vi "FPGA VI_Simulated.vi"() -> ()   [LabVIEW 2015]
uses:
  Types/Injector.Timing.ctl
  Types/Injection.Core.Settings.ctl
  Types/Injection.Global.Settings.ctl
  <vilib>/Platform/TimedLoop/XDataNode/timing_clust.ctl
  <vilib>/Platform/TimedLoop/XDataNode/nitl_modes.ctl
  <vilib>/Platform/TimedLoop/XDataNode/wakeup.ctl
  Types/Injection.Core.Internal.Settings.ctl
  <vilib>/rvi/DataTransferAndStorage/Container/Common/niFpgaContainerGetUniqueNameForEmu.vi
  <vilib>/rvi/DataTransferAndStorage/Container/Common/niFpgaContainerSetEmuInfo.vi
  <vilib>/rvi/eio/common/nirviEmuReportErrorAndStop.vi
  <vilib>/rvi/Emulation/niFpgaGetClockAttributes.vi
  <vilib>/rvi/Emulation/niFpgaSctlEmulationGetInTimedLoop.vi
  <vilib>/rvi/Emulation/niFpgaEmulationReportErrorSimple.vi
  <vilib>/rvi/Memory/Memory_Emulation/nirvimemoryFastEmulation.vi
  <vilib>/rvi/Memory/Memory_Emulation/nirvimemoryEmulation.vi
  <vilib>/rvi/Emulation/niFpgaEmulationIsFPGAContextNoSignature.vi
  <vilib>/rvi/Emulation/niFpgaProcessEmulError.vi
  <vilib>/rvi/errors/nirviReportUnexpectedCaseInternalError (U32).vi
  <vilib>/rvi/Emulation/niFpgaCriticalErrorInLSC.vi
  <vilib>/rvi/DataTransferAndStorage/Container/Common/niFpgaContainerExecOnDevCompGetState.vi
  <vilib>/rvi/errors/niFpgaSetErrorForExecOnDevCompSimple.vi
  <vilib>/rvi/FIFO/Fifo_Resource/nirvififoEmulationSetSize.vi
  <vilib>/rvi/FIFO/Fifo_Resource/nirviFifoEmulationQueueMgr.vi
  <instcachedir>/0/nirviFifoEmulationQueueMgr_E5CAEC123FF24DC58D834DCA3CDAA9B5.lvgen/nirviFifoEmulationQueueMgr_E5CAEC123FF24DC58D834DCA3CDAA9B5_010.vi
  <vilib>/rvi/FIFO/Fifo_Resource/nirvififoEmulationDetermineInputValidOut.vi
  <vilib>/rvi/FIFO/Fifo_Resource/nirvififoEmulationCreateLock.vi
  <vilib>/rvi/FIFO/Fifo_Resource/nirvififoEmulationObtainLock.vi
  <vilib>/rvi/FIFO/Fifo_Resource/nirvififoEmulationReleaseLock.vi
  <vilib>/rvi/occurrence/nirviWaitOnOccurrenceBase.vi
  <vilib>/rvi/errors/nirviReportUnexpectedCaseInternalError.vi
  <vilib>/Utility/error.llb/Clear Errors.vi
  <vilib>/rvi/interface/RandomDataEmulation/niFpgaRandomDataHandleErrors.vi
  <instcachedir>/0/nirviFifoEmulationQueueMgr_E5CAEC123FF24DC58D834DCA3CDAA9B5.lvgen/nirviFifoEmulationQueueMgr_E5CAEC123FF24DC58D834DCA3CDAA9B5_008.vi
  <vilib>/rvi/LocalResourceManager/LocalResourceManager.xnode
  <vilib>/rvi/DataTransferAndStorage/Container/XNode/niFpgaContainer.xnode
  <vilib>/Platform/TimedLoop/XDataNode/XDataNode.xnode
  <vilib>/rvi/FIFO/Fifo_Resource/niFpgaFifoEmulationRefIn.vi
  <vilib>/rvi/interface/RandomDataEmulation/nirviRandomDataFpgaReadWriteTemplate.vi
  <vilib>/Platform/TimedLoop/XDataNode/XDNodeRunTimeDep.lvlib
panel:
  out "Intermediate FIFO Write Timeout":bool
  in  "Settings.Global":T1={"Enable?"=FALSE, "Initial Voltage Threshold"=12.0, "Event Dwell Limit"=2000, "Voltage Gain"=1.0, "Current Gain"=1.0}
  in  "Settings.Index0.Injector0":T2
  in  "Settings.Index1.Injector1":T2
  in  "Settings.Index2.Injector2":T2
  in  "Settings.Index3.Injector3":T2
  in  "Settings.Index4.Injector4":T2
  in  "Settings.Index5.Injector5":T2
  in  "Settings.Timing":T3={"Injector Sample Period (Ticks)"=80}
  out "Acqusition Loop Ticks":u32
  in  "Settings.DMA":cluster{"# of Injectors":u8}={"# of Injectors"=6}
  out "Host DMA Out?":bool
  out "Intermediate Time Out?":bool
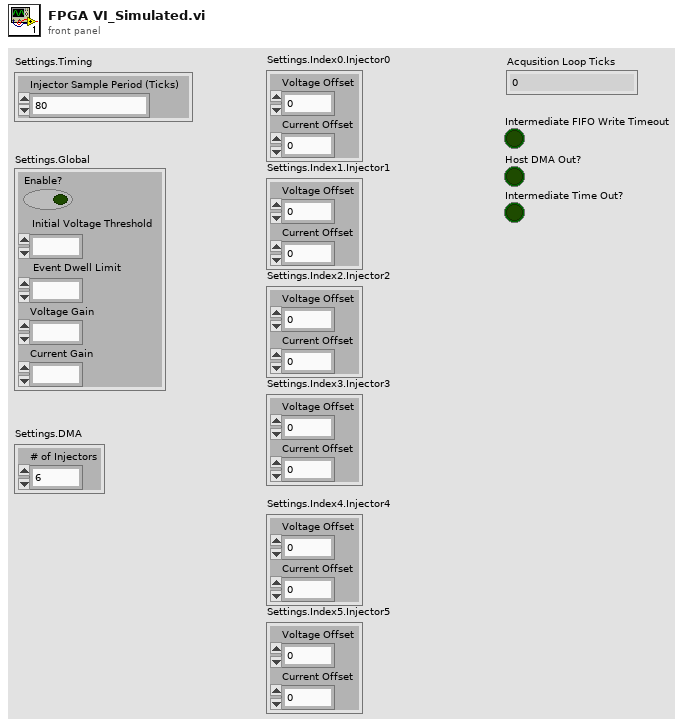
[diagram p1: front panel]
types:
  T1 = typedef "Injection.Global.Settings.ctl" = cluster{"Enable?":bool, "Initial Voltage Threshold":fxp<+/-,32,8>, "Event Dwell Limit":u16, "Voltage Gain":fxp<+/-,32,8>, "Current Gain":fxp<+/-,32,8>}
  T2 = typedef "Injection.Core.Settings.ctl" = cluster{"Voltage Offset":fxp<+/-,32,8>, "Current Offset":fxp<+/-,32,8>}
  T3 = typedef "Injector.Timing.ctl" = cluster{"Injector Sample Period (Ticks)":u32}
  T4 = cluster{"Data.Samples":u32, "Injection.Period":u32, "Injector.Index":u8, "Iteration":u32}
  T5 = enum8{"Wait on Transfer", "Transfer Injector Index", "Transfer # of Samples", "Transfer Injection Period", "Transfer Data Samples"}
  T6 = typedef "XDNodeRunTimeDep.lvlib/timing_clust.ctl" = cluster{"Expected End [f-1]":u64, "Actual End [f-1]":u64, "Finished Late? [f-1]":bool, "Expected End [i-1]":u64, "Actual End [i-1]":u64, "Finished Late? [i-1]":bool, "Expected Start [i]":u64, "Actual Start [i]":u64, "Expected Start [f]":u64, "Actual Start [f]":u64, "Source Name":string, "Structure Name":string, "Period":i64, "Deadline":i64, "Offset":i64, "Start":i64, "Priority":i32, "Timeout":i32, "Mode":T7, "Wakeup Reason":T8, "Error":errorcluster, "Source Type":string, "Secondary Source Type":string, "Global End Time":u64, "Global Start Time":u64, "Frame Duration":u64, "Iteration Duration":u64, "Assigned CPU":i32, "I/O Scan Engine Mode":u32}
  T7 = typedef "XDNodeRunTimeDep.lvlib/nitl_modes.ctl" = enum32{"No Change", "Process missed periods, maintain original phase", "Discard missed periods, maintain original phase", "Process missed periods, ignore original phase", "Discard missed periods, ignore original phase"}
  T8 = typedef "XDNodeRunTimeDep.lvlib/wakeup.ctl" = enum32{"Normal", "Aborted", "Asynchronous wakeup", "Timing source error", "Timed loop error", "Timeout"}
  T9 = typedef "Injection.Core.Internal.Settings.ctl" = cluster{"Data FIFO":refnum<k21>, "Trigger FIFO":refnum<k21>}
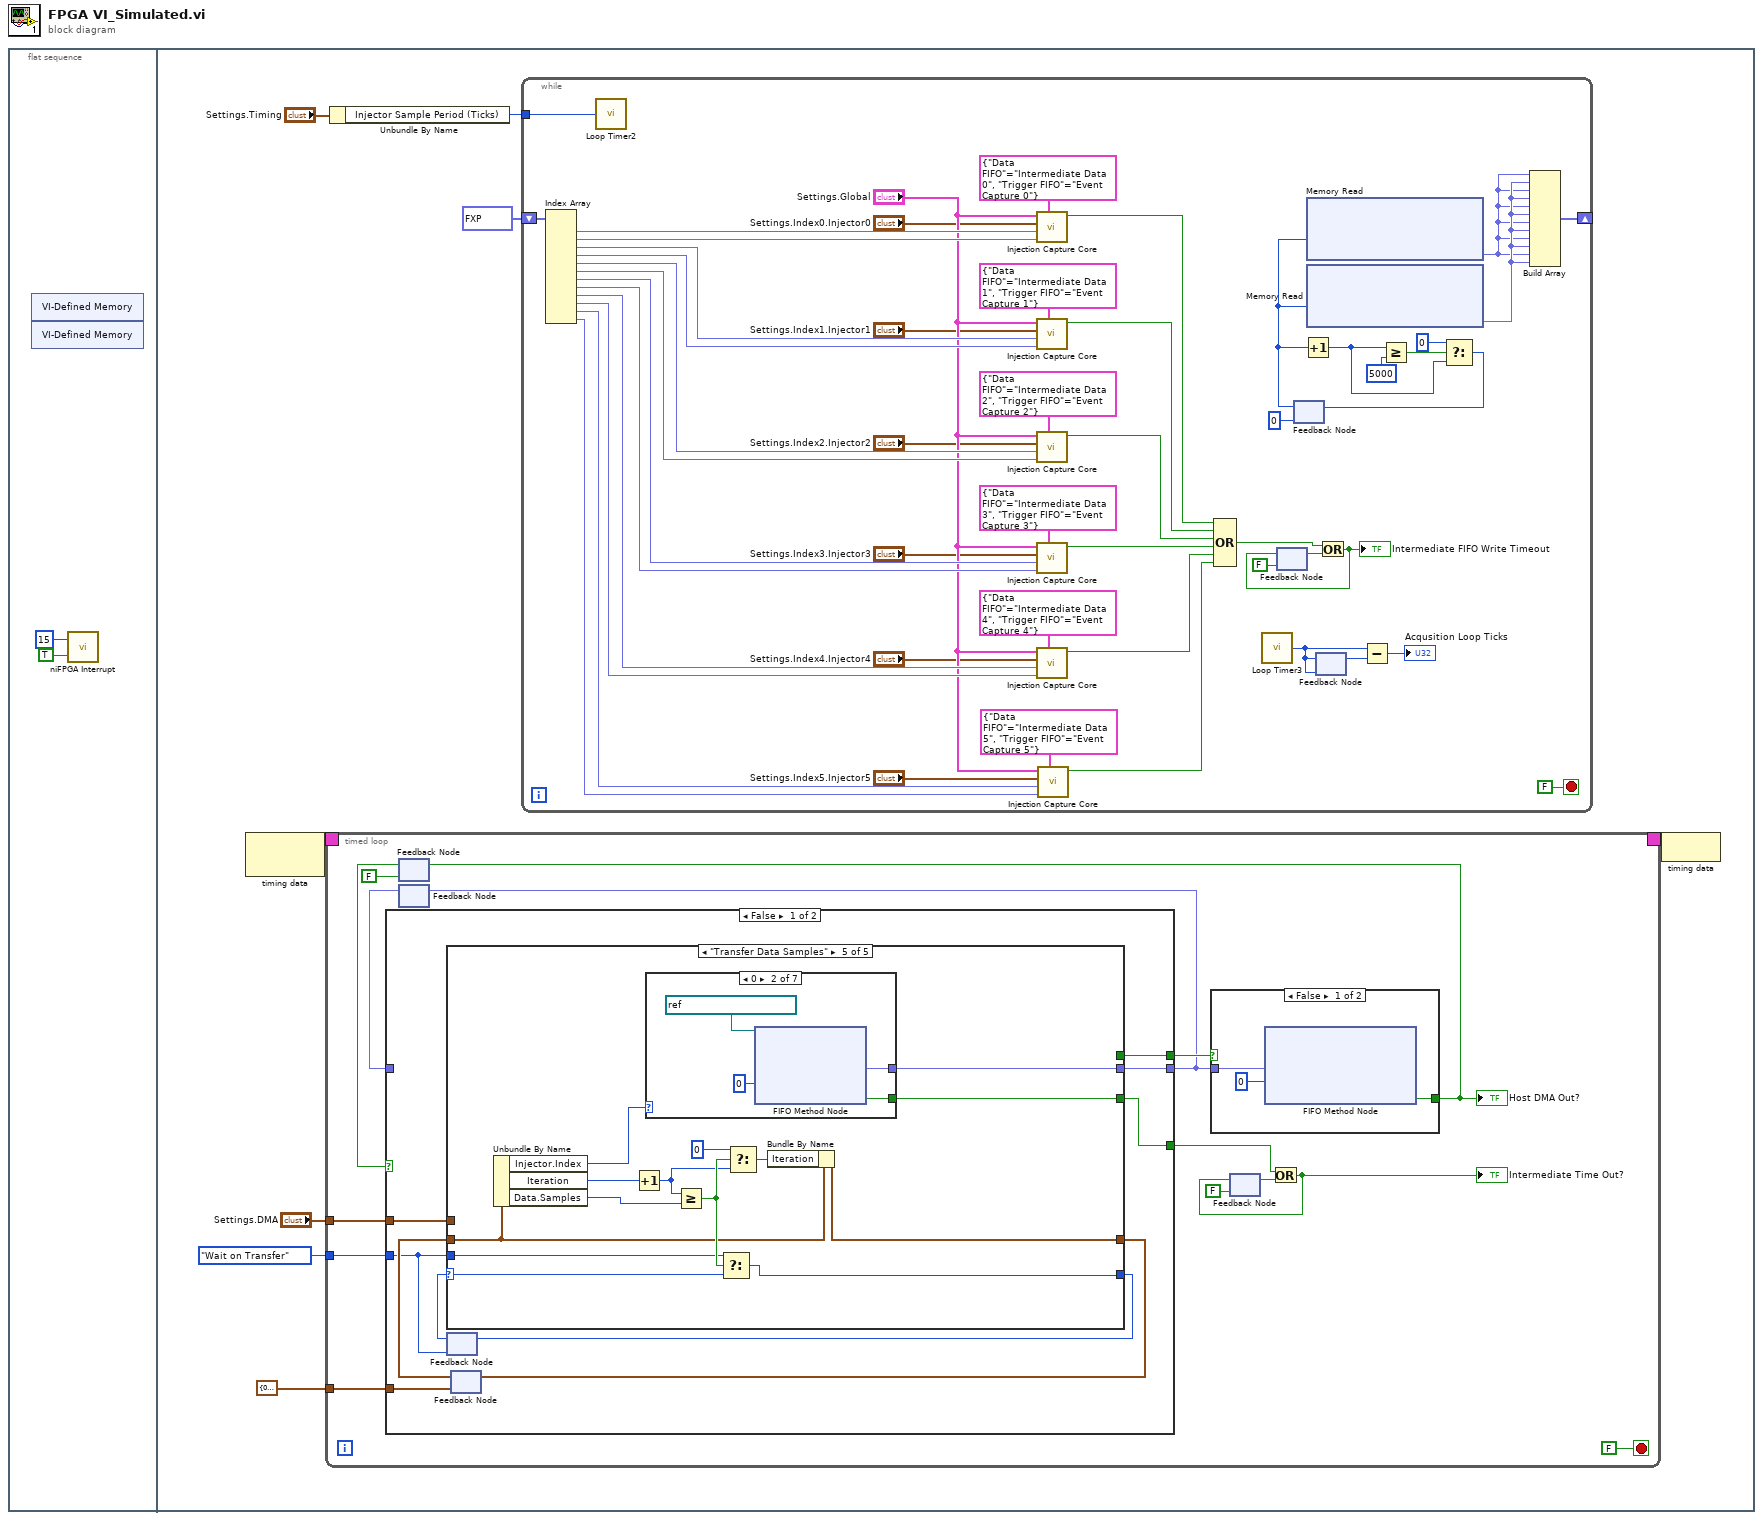
[diagram p0: block diagram]
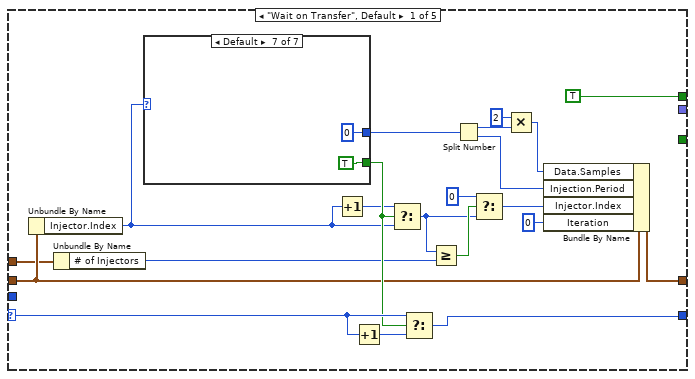
[diagram p2: hidden frame]
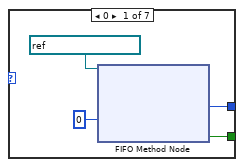
[diagram p3: hidden frame]
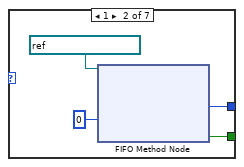
[diagram p4: hidden frame]
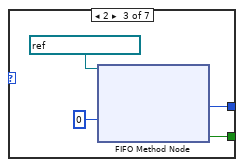
[diagram p5: hidden frame]
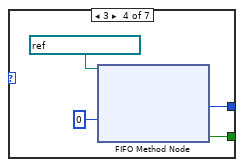
[diagram p6: hidden frame]
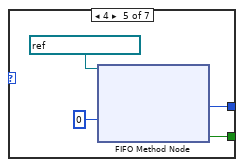
[diagram p7: hidden frame]
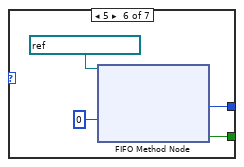
[diagram p8: hidden frame]
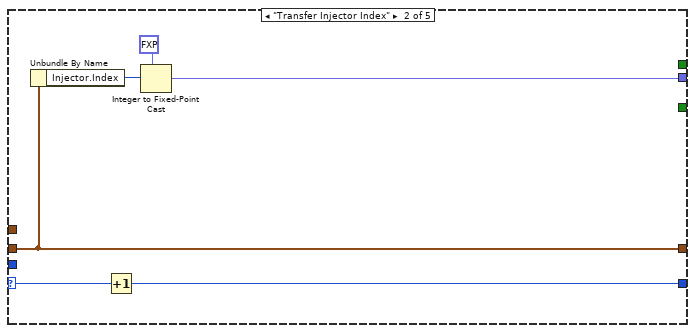
[diagram p9: hidden frame]
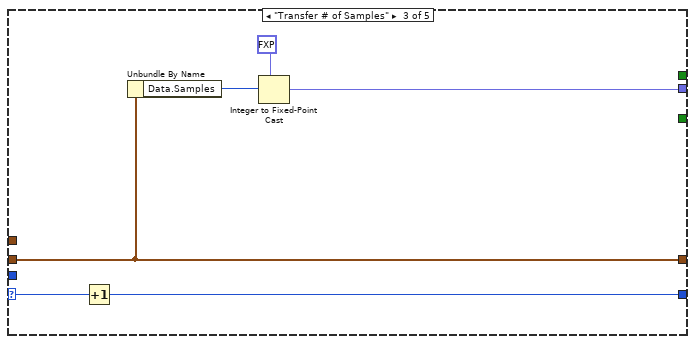
[diagram p10: hidden frame]
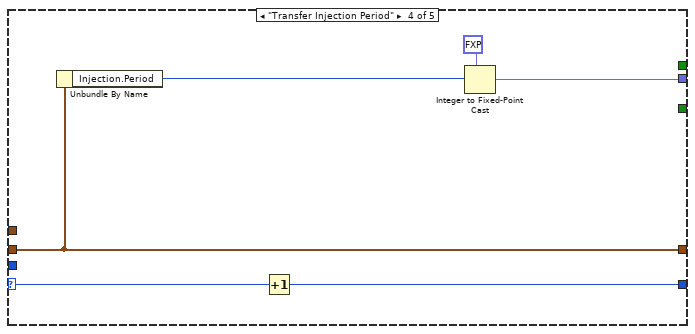
[diagram p11: hidden frame]
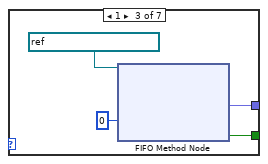
[diagram p13: hidden frame]
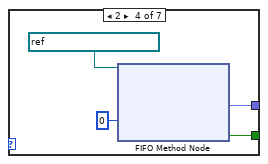
[diagram p14: hidden frame]
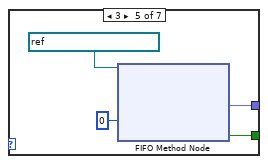
[diagram p15: hidden frame]
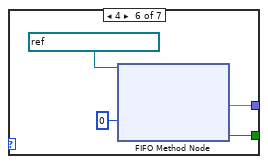
[diagram p16: hidden frame]
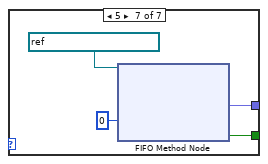
[diagram p17: hidden frame]
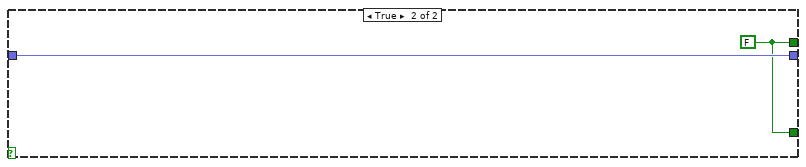
[diagram p18: hidden frame]
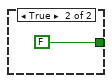
[diagram p19: hidden frame]
diagram:
  n1 = flat-sequence {
    frame #0 {
      n2 = xnode "VI-Defined Memory"() -> ()  [unwired: 1 out]
      n3 = xnode "VI-Defined Memory"() -> ()  [unwired: 1 out]
      n4 = call <vilib>:"niFPGA Interrupt.vi"("Wait Until Cleared (F)"=TRUE, "IRQ Number (0)"=u8 15) -> ()  [unwired: 1 in]
    }
    frame #1 {
      n5 = node-c288() -> (w10:T6)  [unwired: 1 in]
      n6 = timed-loop {
        timing: w10 -> [_]
        timing-out: [_] -> w9
        tunnel: "Settings.DMA" -> [w14]
        tunnel: T5."Wait on Transfer" -> [w13]
        tunnel: T4 {"Data.Samples"=0, "Injection.Period"=0, "Injector.Index"=0, "Iteration"=0} ("Local.Data") -> [w12]
        stop <- FALSE stop-if-true
        n7 = feedback #1(FALSE ("Timed Out?")) -> (w22:bool)
        n8 = feedback #2() -> (w19:fxp<+/-,32,8>)  [unwired: 1 in]
        n9 = case shown="False" w22 {
          tunnel: [w34 w139] -> w20
          tunnel: [w33 w138] -> w24
          tunnel: w13 -> [w26 _]
          tunnel: [w31 w138] -> w15
          tunnel: w14 -> [w30 _]
          tunnel: w12 -> [w27 _]
          tunnel: w19 -> [_ w139]
          frame False {
            n10 = feedback #3(w26) -> (w25:T5)
            n11 = feedback #4(w27) -> (w28:T4)
            n12 = case shown="\"Transfer Data Samples\"" w25 {
              selector: w25 -> [w54 w87 w91 w98 w107]
              tunnel: w28 -> [w45 w84 w89 w95 w105]
              tunnel: [w53 w84 w89 w95 w104] -> w29
              tunnel: [w52 w86 w90 w94 w106] -> w32
              tunnel: [_ w83 w88 w97 w103] -> w34
              tunnel: [TRUE _ _ _ _] -> w33
              tunnel: w26 -> [_ _ _ _ w100]
              tunnel: [_ _ _ _ w102] -> w31
              tunnel: w30 -> [w42 _ _ _ _]
              frame "Wait on Transfer", Default {
                n13 = Unbundle By Name(w45) -> ("Injector.Index"=w44:u8)
                n14 = Unbundle By Name(w42) -> ("# of Injectors"=w41:u8)
                n15 = case shown="Default" w44 {
                  tunnel: [w58 w62 w66 w70 w74 w78 u64 0 ("Element")] -> w40
                  tunnel: [w57 w61 w65 w69 w73 w77 TRUE ("Timed Out?")] -> w50
                  frame 0 {
                    n16 = xnode ("FIFO Method Node")("Timeout"=0, "FIFO In"=refnum<k21> "Event Capture 0") -> ("Element"=w58:u64, "Timed Out?"=w57:bool)  [unwired: 1 out]
                  }
                  frame 1 {
                    n17 = xnode ("FIFO Method Node")("Timeout"=0, "FIFO In"=refnum<k21> "Event Capture 1") -> ("Element"=w62:u64, "Timed Out?"=w61:bool)  [unwired: 1 out]
                  }
                  frame 2 {
                    n18 = xnode ("FIFO Method Node")("Timeout"=0, "FIFO In"=refnum<k21> "Event Capture 2") -> ("Element"=w66:u64, "Timed Out?"=w65:bool)  [unwired: 1 out]
                  }
                  frame 3 {
                    n19 = xnode ("FIFO Method Node")("Timeout"=0, "FIFO In"=refnum<k21> "Event Capture 3") -> ("Element"=w70:u64, "Timed Out?"=w69:bool)  [unwired: 1 out]
                  }
                  frame 4 {
                    n20 = xnode ("FIFO Method Node")("Timeout"=0, "FIFO In"=refnum<k21> "Event Capture 4") -> ("Element"=w74:u64, "Timed Out?"=w73:bool)  [unwired: 1 out]
                  }
                  frame 5 {
                    n21 = xnode ("FIFO Method Node")("Timeout"=0, "FIFO In"=refnum<k21> "Event Capture 5") -> ("Element"=w78:u64, "Timed Out?"=w77:bool)  [unwired: 1 out]
                  }
                  frame Default {
                  }
                }
                n22 = Increment(x=w44) -> (x+1=w49:u8)
                n23 = Increment(x=w54) -> (x+1=w55:T5)
                n24 = Select(t=w49, s=w50, f=w44) -> (s? t:f=w47:u8)
                n25 = Select(t=w54, s=w50, f=w55) -> (s? t:f=w52:T5)
                n26 = Greater Or Equal?(x=w47, y=w41) -> (x >= y?=w48:bool)
                n27 = Split Number(x=w40) -> (hi(x)=w39:u32, lo(x)=w38:u32)
                n28 = Select(t=u8 0, s=w48, f=w47) -> (s? t:f=w43:u8)
                n29 = Multiply(x=u32 2, y=w39) -> (x*y=w36:u32)
                n30 = Bundle By Name(cluster=w45, "Data.Samples"=w36, "Injection.Period"=w38, "Injector.Index"=w43, "Iteration"=u32 0) -> (w53:T4)
              }
              frame "Transfer Injector Index" {
                n31 = Unbundle By Name(w84) -> ("Injector.Index"=w85:u8)
                n32 = Increment(x=w87) -> (x+1=w86:T5)
                n33 = Integer to Fixed-Point Cast(fixed-point type=fxp<+/-,32,8> 0.0, integer=w85) -> (fixed-point=w83:fxp<+/-,32,8>)
              }
              frame "Transfer # of Samples" {
                n34 = Increment(x=w91) -> (x+1=w90:T5)
                n35 = Unbundle By Name(w89) -> ("Data.Samples"=w92:u32)
                n36 = Integer to Fixed-Point Cast(fixed-point type=fxp<+/-,32,8> 0.0, integer=w92) -> (fixed-point=w88:fxp<+/-,32,8>)
              }
              frame "Transfer Injection Period" {
                n37 = Unbundle By Name(w95) -> ("Injection.Period"=w96:u32)
                n38 = Increment(x=w98) -> (x+1=w94:T5)
                n39 = Integer to Fixed-Point Cast(fixed-point type=fxp<+/-,32,8> 0.0, integer=w96) -> (fixed-point=w97:fxp<+/-,32,8>)
              }
              frame "Transfer Data Samples" {
                n40 = Unbundle By Name(w105) -> ("Injector.Index"=w113:u8, "Iteration"=w108:u32, "Data.Samples"=w101:u32)
                n41 = Increment(x=w108) -> (x+1=w110:u32)
                n42 = case shown="0" w113 {
                  tunnel: [_ w116 w120 w124 w128 w132 w136] -> w103
                  tunnel: [_ w115 w119 w123 w127 w131 w135] -> w102
                  frame Default {
                  }
                  frame 0 {
                    n43 = xnode ("FIFO Method Node")("Timeout"=0, "FIFO In"=refnum<k21> "Intermediate Data 0" ("Voltage FIFO")) -> ("Element"=w116:fxp<+/-,32,8>, "Timed Out?"=w115:bool)  [unwired: 1 out]
                  }
                  frame 1 {
                    n44 = xnode ("FIFO Method Node")("Timeout"=0, "FIFO In"=refnum<k21> "Intermediate Data 1" ("Voltage FIFO")) -> ("Element"=w120:fxp<+/-,32,8>, "Timed Out?"=w119:bool)  [unwired: 1 out]
                  }
                  frame 2 {
                    n45 = xnode ("FIFO Method Node")("Timeout"=0, "FIFO In"=refnum<k21> "Intermediate Data 2" ("Voltage FIFO")) -> ("Element"=w124:fxp<+/-,32,8>, "Timed Out?"=w123:bool)  [unwired: 1 out]
                  }
                  frame 3 {
                    n46 = xnode ("FIFO Method Node")("Timeout"=0, "FIFO In"=refnum<k21> "Intermediate Data 3" ("Voltage FIFO")) -> ("Element"=w128:fxp<+/-,32,8>, "Timed Out?"=w127:bool)  [unwired: 1 out]
                  }
                  frame 4 {
                    n47 = xnode ("FIFO Method Node")("Timeout"=0, "FIFO In"=refnum<k21> "Intermediate Data 4" ("Voltage FIFO")) -> ("Element"=w132:fxp<+/-,32,8>, "Timed Out?"=w131:bool)  [unwired: 1 out]
                  }
                  frame 5 {
                    n48 = xnode ("FIFO Method Node")("Timeout"=0, "FIFO In"=refnum<k21> "Intermediate Data 5" ("Voltage FIFO")) -> ("Element"=w136:fxp<+/-,32,8>, "Timed Out?"=w135:bool)  [unwired: 1 out]
                  }
                }
                n49 = Greater Or Equal?(x=w110, y=w101) -> (x >= y?=w112:bool)
                n50 = Select(t=w100, s=w112, f=w107) -> (s? t:f=w106:T5)
                n51 = Select(t=u32 0, s=w112, f=w110) -> (s? t:f=w109:u32)
                n52 = Bundle By Name(cluster=w105, "Iteration"=w109) -> (w104:T4)
              }
            }
            n53 = feedback-in #3(w32) -> ()
            n54 = feedback-in #4(w29) -> ()
          }
          frame True {
            w138 = FALSE
          }
        }
        n55 = feedback-in #2(w20) -> ()
        n56 = case shown="False" w24 {
          tunnel: w20 -> [w141 _]
          tunnel: [w140 FALSE ("Timed Out?")] -> w23
          frame False {
            n57 = xnode ("FIFO Method Node")("Element"=w141, "Timeout"=0) -> ("Timed Out?"=w140:bool)  [unwired: 1 in, 1 out]
          }
          frame True {
          }
        }
        "Host DMA Out?" <- w23
        n58 = feedback-in #1(w23) -> ()
        n59 = feedback #5(FALSE ("Timed Out?")) -> (w17:bool)
        n60 = Or(x=w15, y=w17) -> (x .or. y?=w16:bool)
        "Intermediate Time Out?" <- w16
        n61 = feedback-in #5(w16) -> ()
      }
      n62 = Unbundle By Name("Settings.Timing") -> ("Injector Sample Period (Ticks)"=w3:u32)
      n63 = while {
        shift-right: [w148] -> _
        shift-left: fxp<+/-,24,5>[] [0.0, 0.0, 0.0, 0.0, 0.0, 0.0, 0.0, 0.0, 0.0, 0.0, 0.0, 0.0] -> [w179]
        tunnel: w3 -> [w163]
        stop <- FALSE stop-if-true
        n64 = Index Array(array=w179) -> (element #1=w190:fxp<+/-,24,5>, element #2=w191:fxp<+/-,24,5>, element #3=w188:fxp<+/-,24,5>, element #4=w189:fxp<+/-,24,5>, element #5=w186:fxp<+/-,24,5>, element #6=w187:fxp<+/-,24,5>, element #7=w184:fxp<+/-,24,5>, element #8=w185:fxp<+/-,24,5>, element #9=w182:fxp<+/-,24,5>, element #10=w183:fxp<+/-,24,5>, element #11=w180:fxp<+/-,24,5>, element #12=w181:fxp<+/-,24,5>)  [unwired: 12 in]
        n65 = call "Loop Timer2"("Count(Ticks)"=w163) -> ()  [unwired: 1 out]
        n66 = call "Injection Capture Core.vi"("FIFOs"=T9 {"Data FIFO"="Intermediate Data 0", "Trigger FIFO"="Event Capture 0"} ("InjectorCore.Settings"), "Current (PreScaled)"=w191, "Voltage (PreScaled)"=w190, "Settings.Index<#>.<UserName>"="Settings.Index0.Injector0", "Settings.Global"="Settings.Global") -> ("Intermediate FIFO Timeout?"=w198:bool)  [unwired: 4 in, 2 out]
        n67 = call "Injection Capture Core.vi"("FIFOs"=T9 {"Data FIFO"="Intermediate Data 1", "Trigger FIFO"="Event Capture 1"} ("InjectorCore.Settings"), "Current (PreScaled)"=w189, "Voltage (PreScaled)"=w188, "Settings.Index<#>.<UserName>"="Settings.Index1.Injector1", "Settings.Global"="Settings.Global") -> ("Intermediate FIFO Timeout?"=w197:bool)  [unwired: 4 in, 2 out]
        n68 = call "Injection Capture Core.vi"("FIFOs"=T9 {"Data FIFO"="Intermediate Data 2", "Trigger FIFO"="Event Capture 2"} ("InjectorCore.Settings"), "Current (PreScaled)"=w187, "Voltage (PreScaled)"=w186, "Settings.Index<#>.<UserName>"="Settings.Index2.Injector2", "Settings.Global"="Settings.Global") -> ("Intermediate FIFO Timeout?"=w196:bool)  [unwired: 4 in, 2 out]
        n69 = call "Injection Capture Core.vi"("FIFOs"=T9 {"Data FIFO"="Intermediate Data 3", "Trigger FIFO"="Event Capture 3"} ("InjectorCore.Settings"), "Current (PreScaled)"=w185, "Voltage (PreScaled)"=w184, "Settings.Index<#>.<UserName>"="Settings.Index3.Injector3", "Settings.Global"="Settings.Global") -> ("Intermediate FIFO Timeout?"=w195:bool)  [unwired: 4 in, 2 out]
        n70 = call "Injection Capture Core.vi"("FIFOs"=T9 {"Data FIFO"="Intermediate Data 4", "Trigger FIFO"="Event Capture 4"} ("InjectorCore.Settings"), "Current (PreScaled)"=w183, "Voltage (PreScaled)"=w182, "Settings.Index<#>.<UserName>"="Settings.Index4.Injector4", "Settings.Global"="Settings.Global") -> ("Intermediate FIFO Timeout?"=w194:bool)  [unwired: 4 in, 2 out]
        n71 = call "Injection Capture Core.vi"("FIFOs"=T9 {"Data FIFO"="Intermediate Data 5", "Trigger FIFO"="Event Capture 5"} ("InjectorCore.Settings"), "Current (PreScaled)"=w181, "Voltage (PreScaled)"=w180, "Settings.Index<#>.<UserName>"="Settings.Index5.Injector5", "Settings.Global"="Settings.Global") -> ("Intermediate FIFO Timeout?"=w193:bool)  [unwired: 4 in, 2 out]
        n72 = Compound Arithmetic op=OR(w198, w197, w196, w195, w194, w193) -> (w168:bool)
        n73 = call "Loop Timer3"() -> ("Tick Count(Ticks)"=w164:u32)  [unwired: 1 in]
        n74 = feedback #6(FALSE ("Timed Out?")) -> (w169:bool)
        n75 = feedback #7(u32 0 ("Address")) -> (w155:u32)
        n76 = Increment(x=w155) -> (x+1=w151:u32)
        n77 = xnode ("Memory Read")("Address"=w155) -> ("Data"=w156:fxp<+/-,24,5>)  [unwired: 1 in, 1 out]
        n78 = xnode ("Memory Read")("Address"=w155) -> ("Data"=w157:fxp<+/-,24,5>)  [unwired: 1 in, 1 out]
        n79 = feedback-in #8(w164) -> ()
        n80 = feedback #8(w164) -> (w166:u32)
        n81 = Or(x=w168, y=w169) -> (x .or. y?=w167:bool)
        "Intermediate FIFO Write Timeout" <- w167
        n82 = feedback-in #6(w167) -> ()
        n83 = Subtract(x=w164, y=w166) -> (x-y=→"Acqusition Loop Ticks":u32)
        n84 = Greater Or Equal?(x=w151, y=u32 5000) -> (x >= y?=w150:bool)
        n85 = Select(t=u32 0, s=w150, f=w151) -> (s? t:f=w153:u32)
        n86 = feedback-in #7(w153) -> ()
        n87 = Build Array(w156, w157, w156, w157, w156, w157, w156, w157, w156, w157, w156, w157) -> (w148:fxp<+/-,24,5>[])
      }
      n88 = node-c288(w9) -> ()
    }
  }
